vi "Events_Composer.vi"(8 "hearbeat":bool, 10 "time":u32=17041, 11 "responsein":string="{\"result\":[[\"intout\",\"stringout\",\"booleanout\",\"doubleout\",\"time\",\"arrayout\"],[0,\"hola\",false,0.000000,17.000000,[0.000000,0.000000]]]}") -> (3 "responseout":string="{\"result\":[[\"intout\",\"stringout\",\"booleanout\",\"doubleout\",\"time\",\"arrayout\"],[0,\"hola\",false,0.000000,17.000000,[0.000000,0.000000]]]}")   [LabVIEW 2015]
doc: "Definition of all events sent by the SSE server to the clients"
panel:
  in  "periodic":bool=TRUE
  # "Events"
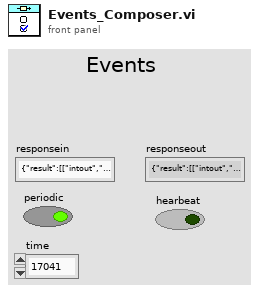
[diagram p1: front panel]
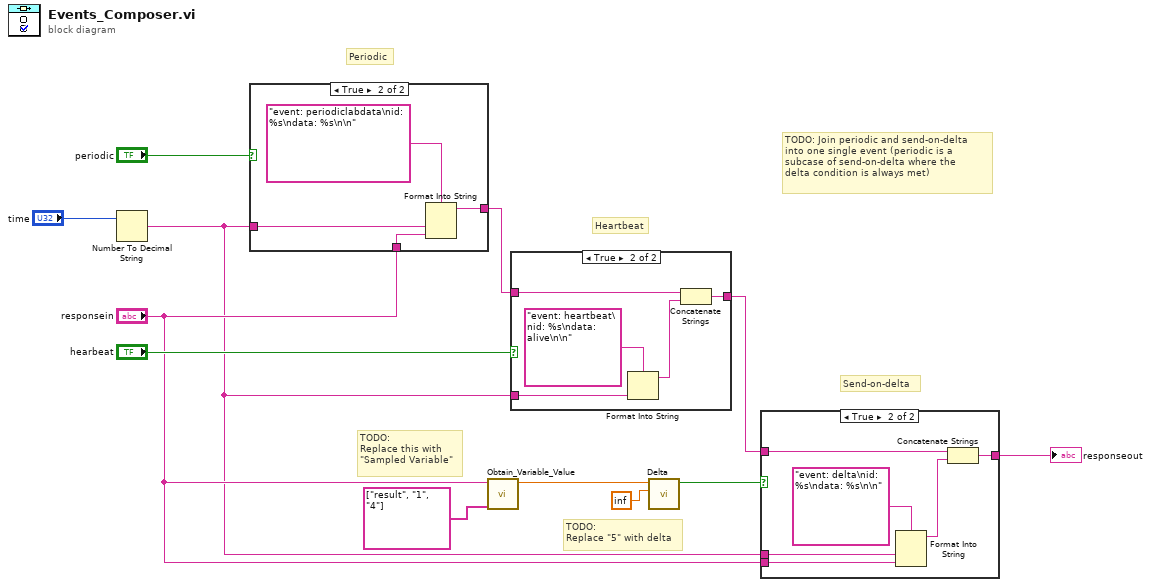
[diagram p0: block diagram]
diagram:
  # "TODO:\nReplace \"5\" with delta"
  # "TODO: Join periodic and send-on-delta\ninto one single event (periodic is a\nsubcase of send-on-delta where the \ndelta condition is always met)"
  # "Send-on-delta"
  # "Heartbeat"
  # "Periodic"
  # "TODO: \nReplace this with\n\"Sampled Variable\""
  n1 = Number To Decimal String(number="time") -> (decimal integer string=w3:string)  [unwired: 1 in]
  n2 = case shown="True" "periodic" {
    tunnel: [w13 w14] -> w5
    tunnel: w3 -> [_ w16]
    tunnel: "responsein" -> [w13 w15]
    frame False {
    }
    frame True {
      n3 = Format Into String(format string="event: periodiclabdata\nid: %s\ndata: %s\n\n", w16, w15) -> (resulting string=w14:string)  [unwired: 2 in, 1 out]
    }
  }
  n4 = call "Obtain_Variable_Value.vi"("path"=string[] ["result", "1", "4"], "JSON result"="responsein") -> ("currentValue"=w10:dbl)  [unwired: 8 in]
  n5 = case shown="True" "hearbeat" {
    tunnel: [w18 w23] -> w7
    tunnel: w5 -> [w18 w22]
    tunnel: w3 -> [_ w19]
    frame False {
    }
    frame True {
      n6 = Format Into String(format string="event: heartbeat\nid: %s\ndata: alive\n\n", w19) -> (resulting string=w20:string)  [unwired: 2 in, 1 out]
      n7 = Concatenate Strings(w22, w20) -> (w23:string)
    }
  }
  n8 = call "Delta.vi"("currentValue"=w10, "delta"=inf) -> ("triggerEvent"=w2:bool)  [unwired: 8 in]
  n9 = case shown="True" w2 {
    tunnel: [w24 w27] -> w8
    tunnel: w7 -> [w24 w26]
    tunnel: "responsein" -> [_ w29]
    tunnel: w3 -> [_ w28]
    frame False {
    }
    frame True {
      n10 = Format Into String(format string="event: delta\nid: %s\ndata: %s\n\n", w28, w29) -> (resulting string=w25:string)  [unwired: 2 in, 1 out]
      n11 = Concatenate Strings(w26, w25) -> (w27:string)
    }
  }
  "responseout" <- w8
